vi "test_ThreeSessTwoPinThreeInstrTwoSiteReservation_CallNiDmmGetConnections1PinMConnections_ReturnsTwoConnections.vi"(8 "error in":errorcluster) -> (0 "error out":errorcluster, 2 "result":string, 3 "pass":bool)   [LabVIEW 2020, in "MeasurementServerTests.lvlib"]
uses:
  MeasurementServerTests.lvlib
  Runtime/Clients/Session Management V1/Session Reservation/Connection.ctl
  Runtime/Clients/Session Management V1/Session Reservation/Session Reservation.lvclass
  03fc85e1-696b-4ece-a78b-f41470766ac0.vi
  a536e905-e99b-4ce6-9f7b-add65bd26abc.vi
  Runtime/Sessions/niDMM/Connection with Session.ctl
  Runtime/Sessions/niDMM/NI Session Management niDMM.lvlib
  Runtime/Sessions/niDMM/Get Connections - 1Pin MConn.vi
  d0d223bc-79f6-43e2-af9c-51012d710bfe.vi
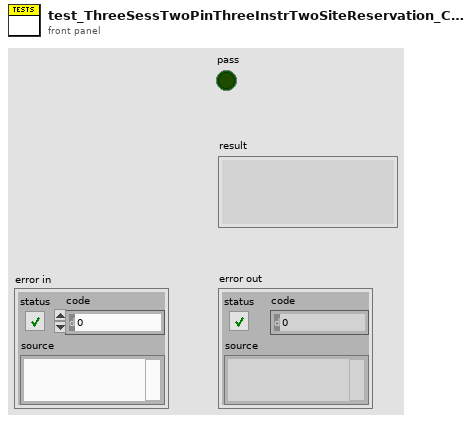
[diagram p1: front panel]
types:
  T1 = typedef "NI Session Management niDMM.lvlib/Connection with Session.ctl" = cluster{"connection":T2, "session":refnum<k15>}
  T2 = typedef "NI Session Management V1 Client.lvlib/Session Reservation.lvclass/Connection.ctl" = cluster{"pin or relay name":string, "site":i32, "instrument type id":string, "channel":string}
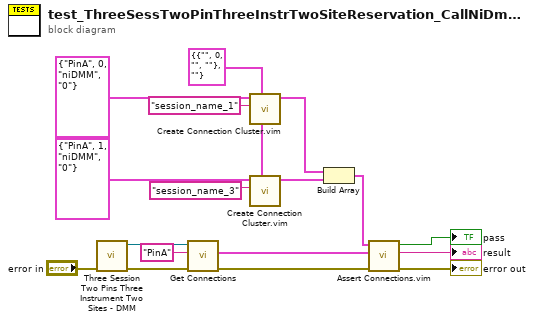
[diagram p0: block diagram]
diagram:
  w10 = T1 {"connection"={"pin or relay name"="", "site"=0, "instrument type id"="", "channel"=""}, "session"=""} ("connection with session")
  n1 = call "Three Session Two Pins Three Instrument Two Sites - DMM.vi"("error in"="error in") -> ("error out"=w3:errorcluster, "session reservation out"=w4:refnum<class "Session Reservation.lvclass">)  [unwired: 9 in]
  n2 = call-poly "Get Connections.vi"("error in"=w3, "pin or relay name"="PinA", "session reservation in"=w4) -> ("error out"=w2:errorcluster, "connections"=w8:T1[])  [unwired: 6 in, 1 out]
  n3 = call "Create Connection Cluster.vim"("connection type"=w10, "session in"="session_name_1", "hardware independent connection in"=T2 {"pin or relay name"="PinA", "site"=0, "instrument type id"="niDMM", "channel"="0"} ("connection")) -> ("connection out"=w13:T1)  [unwired: 8 in]
  n4 = call "Create Connection Cluster.vim"("connection type"=w10, "session in"="session_name_3", "hardware independent connection in"=T2 {"pin or relay name"="PinA", "site"=1, "instrument type id"="niDMM", "channel"="0"} ("connection")) -> ("connection out"=w12:T1)  [unwired: 8 in]
  n5 = Build Array(w13, w12) -> (w11:T1[])
  n6 = call "Assert Connections.vim"("error in"=w2, "actual connections"=w8, "expected connections"=w11) -> ("error out"=→"error out":errorcluster, "result"=→"result":string, "pass"=→"pass":bool)  [unwired: 6 in]
